vi "create test channels.vi"() -> (0 "error out":errorcluster, 1 "channel names":string[](array[string]), 2 "group names":string[](array[string]), 3 "TDMS datalogger configuration out":refnum<class "TDMS datalogger configuration.lvclass">, 4 "File Property Names":string[](array[string])=["FileName", "UserName"], 5 "chans":refnum<class "TBM channel.lvclass">[](array[class]), 6 "File Property Values":string[](array[string])=["File1", "User"], 7 "Channel Types":T2[](array[typedef]), 8 "Lines":T1(array[cluster]))   [LabVIEW 2015, in "tdms logger tests.lvlib"]
uses:
  tdms logger tests.lvlib
  <vilib>/NI/Tag Bus Module Framework/channel/TBM channel.lvclass
  configuration/TDMS datalogger configuration.lvclass
  <vilib>/NI/Tag Bus/tag/Data Type.ctl
  <vilib>/NI/LogRotate/options.ctl
  <vilib>/NI/Tag Bus Module Framework/channel/channel classification.ctl
  <vilib>/NI/Tag Bus/tag/tag descriptor.lvclass/tag descriptor.ctl
  configuration/TDMS datalogger configuration.lvclass/TDMS datalogger configuration.ctl
  configuration/Write queue size.vi
  configuration/Write scans per write.vi
  configuration/Write backup directory.vi
  configuration/Write log directory.vi
  configuration/Write log name.vi
  configuration/Write add enable channel.vi
  configuration/Write logrotate_options.vi
  <vilib>/NI/Tag Bus/tag/default value polymorphs/write default value String.vi
  <vilib>/NI/Configuration Framework/serializable configuration/NISE_CEF_serializable configuration.lvclass
  <vilib>/NI/LogRotate/LogRotate.lvclass
  <vilib>/NI/Tag Bus/tag/tag descriptor.lvclass
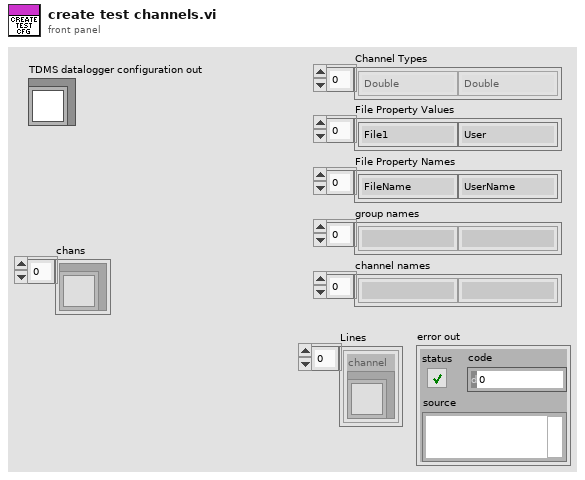
[diagram p1: front panel]
types:
  T1 = cluster{"channel":refnum<class "TBM channel.lvclass">}[]
  T2 = typedef "tag bus.lvlib/tag descriptor.lvclass/Data Type.ctl" = enum16{"Double", "Single", "I64", "I32", "I16", "I8", "U64", "U32", "U16", "U8", "Boolean", "String", "Array of Double", "Array of Single", "Array of I64", "Array of I32", "Array of I16", "Array of I8", "Array of U64", "Array of U32", "Array of U16", "Array of U8", "Array of Boolean", "Array of String"}
  T3 = typedef "TBM channel.lvclass/channel classification.ctl" = enum16{"input data", "output data", "processing parameter", "processing result"}
  T4 = typedef "LogRotate.lvclass/options.ctl" = cluster{"max file size (bytes)":i64, "rotate count":u32, "max age (days)":dbl, "No archive dir":bool, "Archive dir":path}
  T5 = cluster{"channel":refnum<class "TBM channel.lvclass">}
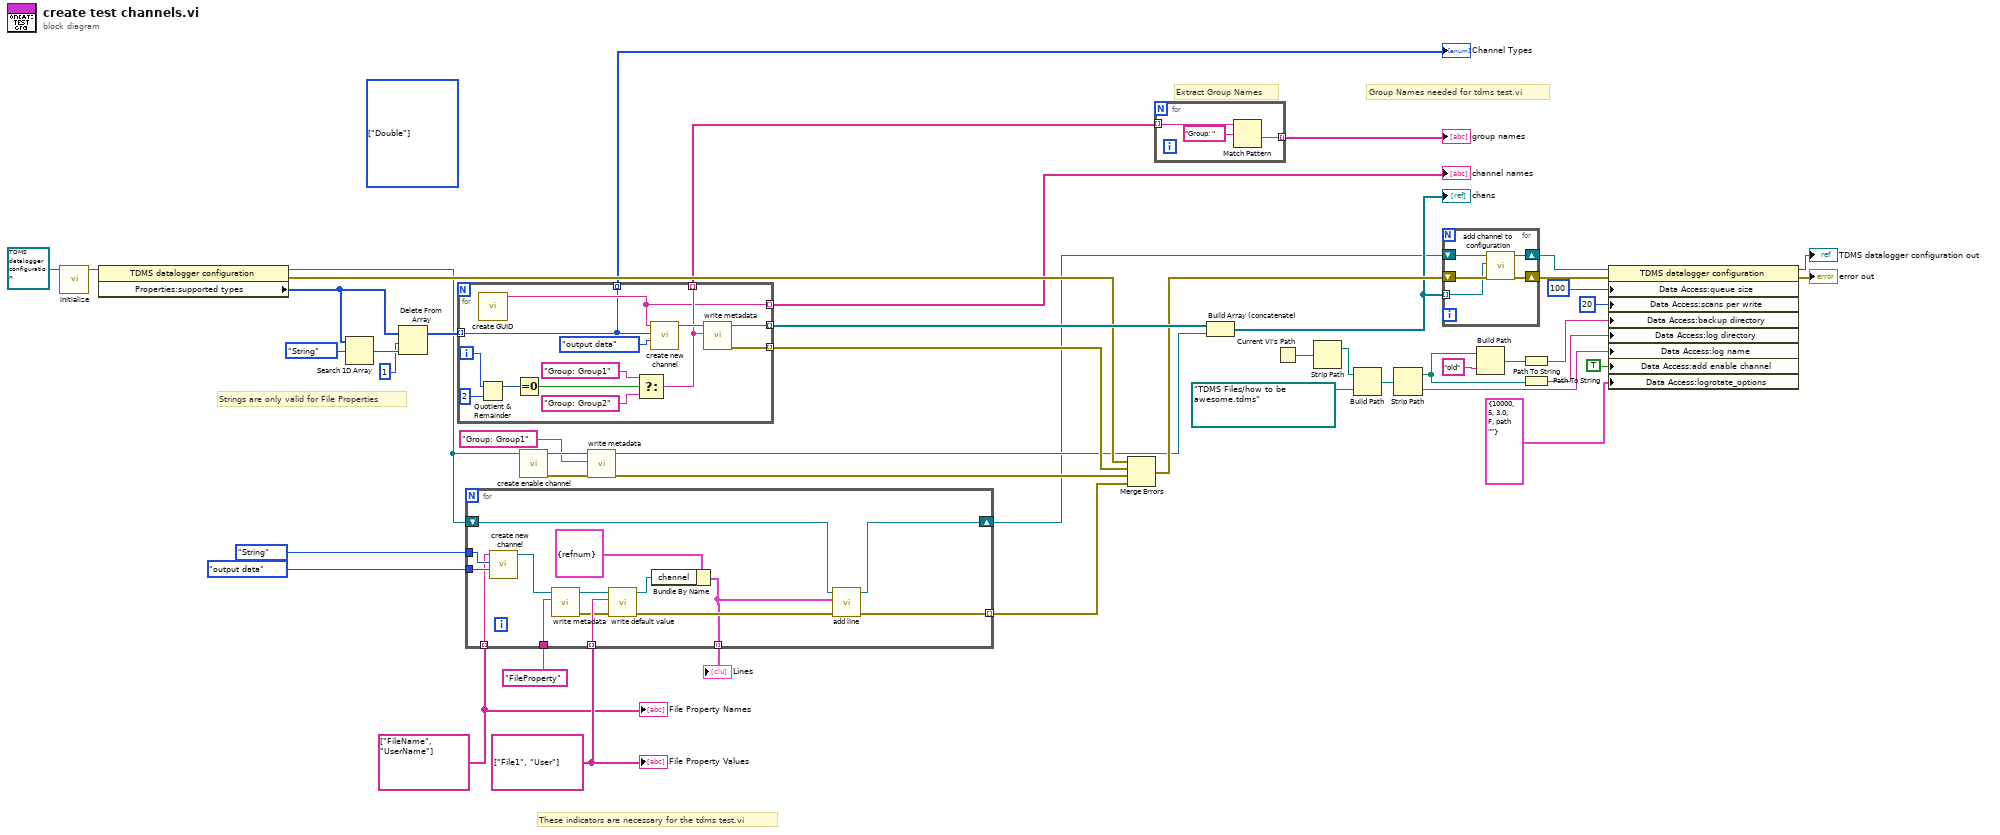
[diagram p0: block diagram]
diagram:
  (unwired) T2[] [enum."Double"] items=["Double", "Single", "I64", "I32", "I16", "I8", "U64", "U32", "U16", "U8", "Boolean", "String", "Array of Double", "Array of Single", "Array of I64", "Array of I32", "Array of I16", "Array of I8", "Array of U64", "Array of U32", "Array of U16", "Array of U8", "Array of Boolean", "Array of String"] ("Properties:supported types")
  w18 = string[] ["File1", "User"] ("channel name")
  w17 = string[] ["FileName", "UserName"] ("channel name")
  # "Strings are only valid for File Properties"
  # "Extract Group Names"
  # "Group Names needed for tdms test.vi"
  # "These indicators are necessary for the tdms test.vi"
  n1 = call <vilib>:"initialize.vi"("configuration in"=refnum<class "TDMS datalogger configuration.lvclass"> refnum ("TDMS datalogger configuration")) -> ("configuration out"=w45:refnum<class "TDMS datalogger configuration.lvclass">)  [unwired: 8 in, 2 out]
  n2 = property class="TDMS datalogger configuration"(reference=w45) -> (reference out=w3:refnum<class "TDMS datalogger configuration.lvclass">, error out=w47:errorcluster, "Properties:supported types"=w8:T2[])  [unwired: 1 in]
  n3 = Search 1D Array(1D array=w8, element=Data_Type."String") -> (index of element=w9:i32)  [unwired: 1 in]
  n4 = Delete From Array(array=w8, length=1, index=w9) -> (array with subset deleted=w5:T2[])  [unwired: 1 out]
  n5 = for {
    tunnel: [w59] -> w48 mode=indexing
    tunnel: w5 -> [w49] mode=indexing
    tunnel: [w50] -> w44 mode=indexing
    tunnel: [w58] -> w24 mode=indexing
    tunnel: [w52] -> w14 mode=indexing
    tunnel: [w49] -> w6 mode=indexing
    i -> [w51]
    n6 = call <vilib>:"create GUID.vi"() -> ("uuid"=w50:string)  [unwired: 10 in, 1 out]
    n7 = Quotient & Remainder(x=w51, y=2) -> (x-y*floor(x/y)=w54:i32)  [unwired: 1 out]
    n8 = Equal To 0?(x=w54) -> (x = 0?=w53:bool)
    n9 = Select(t="Group: Group1", s=w53, f="Group: Group2") -> (s? t:f=w52:string)
    n10 = call <vilib>:"create new channel.vi"("channel classification"=channel_classification."output data", "data type"=w49, "channel name"=w50) -> ("channel"=w60:refnum<class "TBM channel.lvclass">)  [unwired: 8 in]
    n11 = call <vilib>:"write metadata.vi"("metadata"=w52, "system tag in"=w60) -> ("error out"=w58:errorcluster, "system tag out"=w59:refnum<class "TBM channel.lvclass">)  [unwired: 8 in]
  }
  "channel names" <- w44
  "Channel Types" <- w6
  n12 = for {
    tunnel: "FileProperty" ("metadata") -> [w76]
    tunnel: w18 -> [w75] mode=indexing
    tunnel: channel_classification."output data" ("channel classification") -> [w72]
    tunnel: Data_Type."String" ("data type") -> [w71]
    tunnel: w17 -> [w70] mode=indexing
    tunnel: [w63] -> w16 mode=indexing
    shift-right: [w65] -> w2
    shift-left: w3 -> [w66]
    tunnel: [w62] -> w1 mode=indexing
    n13 = call <vilib>:"create new channel.vi"("channel classification"=w72, "data type"=w71, "channel name"=w70) -> ("channel"=w73:refnum<class "TBM channel.lvclass">)  [unwired: 8 in]
    n14 = call <vilib>:"write metadata.vi"("metadata"=w76, "system tag in"=w73) -> ("error out"=w74:errorcluster, "system tag out"=w69:refnum<class "TBM channel.lvclass">)  [unwired: 8 in]
    n15 = call-poly <vilib>:"write default value.vi"("error in"=w74, "default value"=w75, "system tag in"=w69) -> ("error out"=w64:errorcluster, "system tag out"=w67:refnum<class "TBM channel.lvclass">)  [unwired: 7 in]
    n16 = Bundle By Name(cluster=T5 {"channel"=refnum} ("Line"), "channel"=w67) -> (w62:T5)
    n17 = call "add line.vi"("error in"=w64, "Line"=w62, "TDMS datalogger configuration in"=w66) -> ("error out"=w63:errorcluster, "TDMS datalogger configuration out"=w65:refnum<class "TDMS datalogger configuration.lvclass">)  [unwired: 6 in, 1 out]
  }
  "Lines" <- w1
  n18 = call "create enable channel.vi"("TDMS datalogger configuration"=w3) -> ("error out"=w22:errorcluster, "enable channel"=w23:refnum<class "TBM channel.lvclass">)  [unwired: 8 in, 1 out]
  n19 = call <vilib>:"write metadata.vi"("error in"=w22, "metadata"="Group: Group1", "system tag in"=w23) -> ("error out"=w15:errorcluster, "system tag out"=w12:refnum<class "TBM channel.lvclass">)  [unwired: 7 in]
  n20 = Merge Errors(w47, w24, w15, w16) -> (w25:errorcluster)
  n21 = for {
    tunnel: w14 -> [w79] mode=indexing
    tunnel: [w77] -> w11 mode=indexing
    n22 = Match Pattern(string=w79, regular expression="Group: " ("search string/char (-)")) -> (after substring=w77:string)  [unwired: 1 in, 3 out]
  }
  "group names" <- w11
  n23 = Build Array (concatenate)(w48, w12) -> (w13:refnum<class "TBM channel.lvclass">[])
  "chans" <- w13
  n24 = Current VI's Path() -> (path=w33:path)
  n25 = Strip Path(path=w33) -> (stripped path=w32:path)  [unwired: 1 out]
  n26 = Build Path(base path=w32, name or relative path=path "TDMS Files/how to be awesome.tdms" ("output file path")) -> (appended path=w34:path)
  n27 = Strip Path(path=w34) -> (stripped path=w29:path, name=w31:string)
  n28 = for {
    shift-right: [w83] -> w41
    shift-left: w2 -> [w84]
    shift-right: [w81] -> w38
    shift-left: w25 -> [w82]
    tunnel: w13 -> [w80] mode=indexing
    n29 = call "add channel to configuration.vi"("error in"=w82, "TBM channel in"=w80, "TDMS datalogger configuration in"=w84) -> ("error out"=w81:errorcluster, "TDMS datalogger configuration out"=w83:refnum<class "TDMS datalogger configuration.lvclass">)  [unwired: 7 in]
  }
  n30 = Build Path(base path=w29, name or relative path="old") -> (appended path=w28:path)
  n31 = Path To String(path=w28) -> (string=w37:string)
  n32 = Path To String(path=w29) -> (string=w36:string)
  n33 = property class="TDMS datalogger configuration"(reference=w41, error in=w38, "Data Access:queue size"=100 ("queue size"), "Data Access:scans per write"=20 ("scans per write"), "Data Access:backup directory"=w37, "Data Access:log directory"=w36, "Data Access:log name"=w31, "Data Access:add enable channel"=TRUE ("add enable channel"), "Data Access:logrotate_options"=T4 {"max file size (bytes)"=10000, "rotate count"=5, "max age (days)"=3.0, "No archive dir"=FALSE, "Archive dir"=path ""} ("logrotate_options")) -> (reference out=→"TDMS datalogger configuration out":refnum<class "TDMS datalogger configuration.lvclass">, error out=→"error out":errorcluster)
  "File Property Values" <- w18
  "File Property Names" <- w17
